vi "AUTOFLIM_Align.vi"(0 "Y Scan Center":dbl, 1 "X Scan Center":dbl, 2 "System no.":i32, 5 "Scan Termination":T1(ring), 7 "X":dbl, 9 "Y":dbl, 11 "error in (no error)":errorcluster, 12 "Z":dbl) -> (3 "Mesh out":dbl, 4 "Numeric 2":dbl, 6 "Numeric":dbl, 8 "Alignment Graph":dbl[][](array[numeric]), 10 "3D Line Graph":refnum<class "Base Datatype.lvclass">[](array[class]), 15 "error out":errorcluster)   [LabVIEW 2023]
uses:
  <vilib>/Native 3D Graph/classes/Base Datatype.lvclass
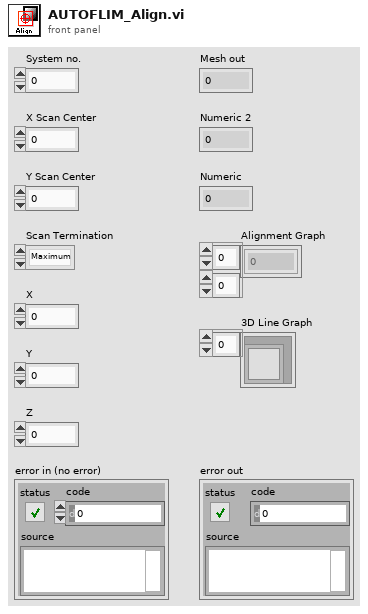
[diagram p1: front panel]
types:
  T1 = enum16{"Maximum", "End Position", "Center of scan"}
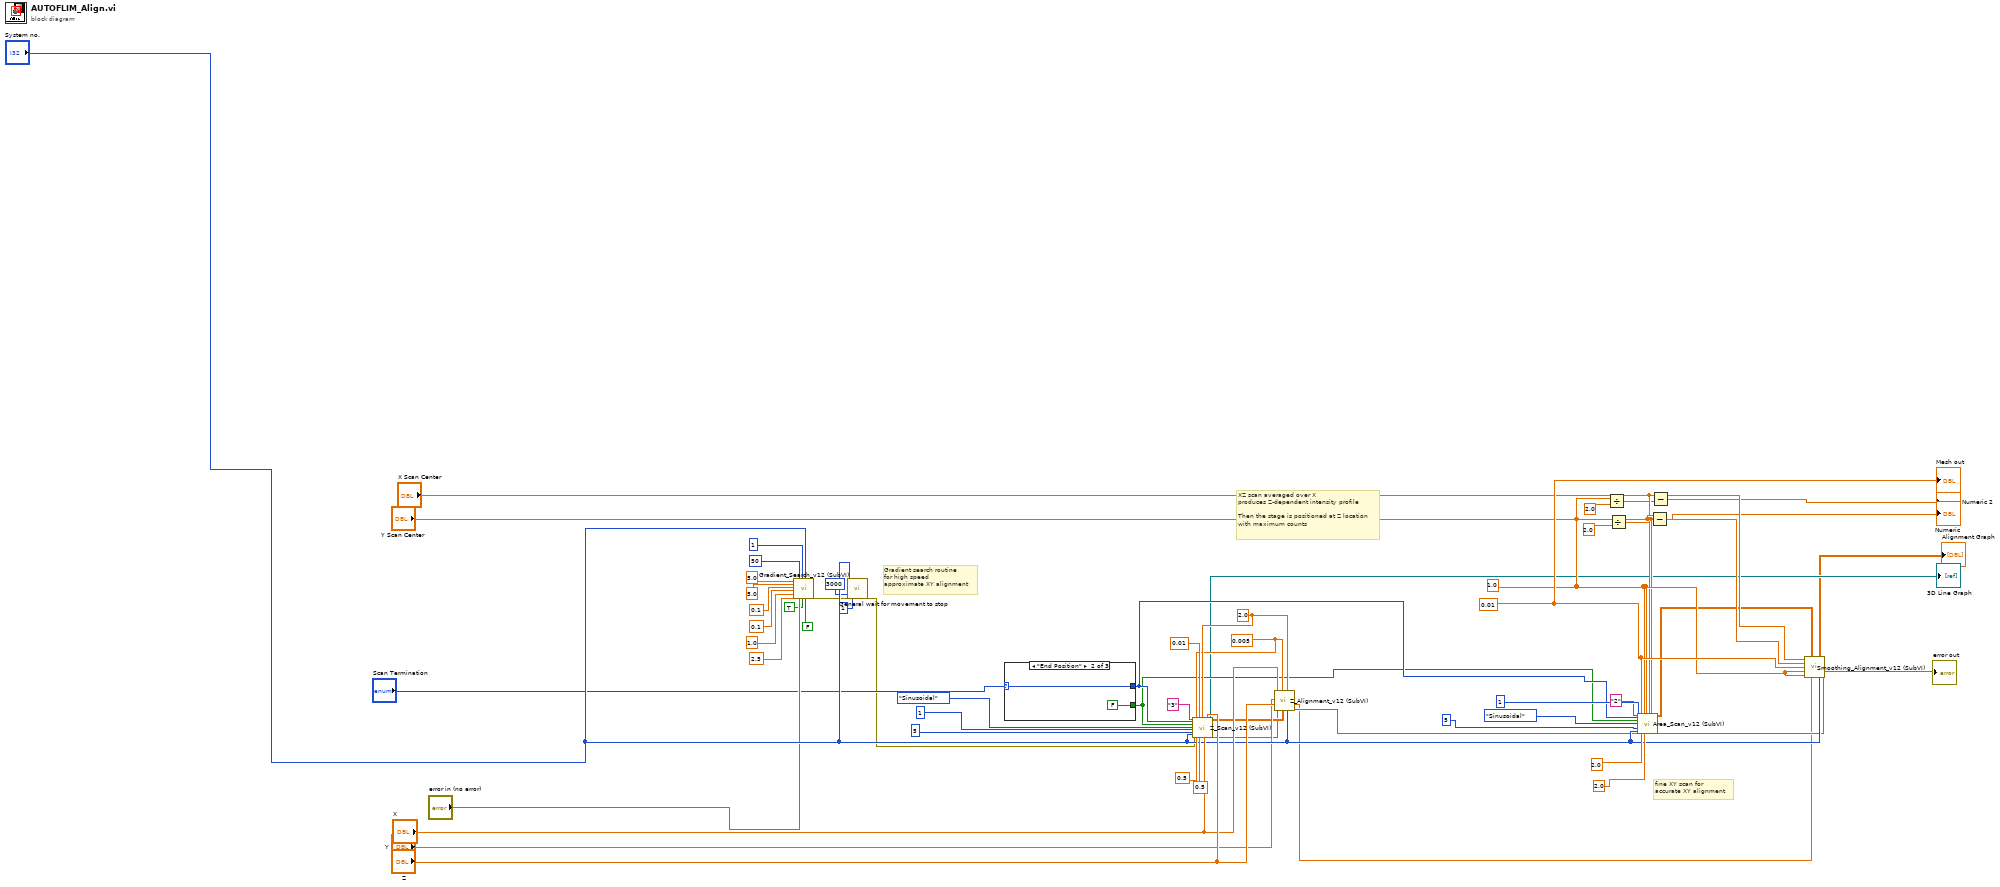
[diagram p0: block diagram]
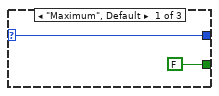
[diagram p2: hidden frame]
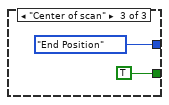
[diagram p3: hidden frame]
diagram:
  w54 = 0.01 ("Mesh in")
  w53 = 1.0 ("X Scan Range")
  w47 = 0.005 ("Z Mesh")
  w48 = 2.0 ("Z range")
  # "fine XY scan for\naccurate XY alignment"
  # "XZ scan averaged over X\nproduces Z-dependent intensity profile\n\nThen the stage is positioned at Z location\nwith maximum counts"
  # "Gradient search routine\nfor high speed\napproximate XY alignment"
  n1 = call "Gradient_Search_v12 (SubVI).vi"("Speed factor"=5.0, "Max velocity"=5.0, "ML"=0.1, "Min Radius"=0.1, "Max Radius"=1.0, "GS Frequency"=2.5, "Max. dir. changes"=50, "error in (no error)"="error in (no error)", "Analog Input"=1, "Run?"=TRUE, "System no."="System no.", "Tracking"=FALSE) -> ("error out"=w10:errorcluster)  [unwired: 7 in]
  n2 = call "General wait for movement to stop.vi"("System no."="System no.", "Additional wait time, ms"=3000, "error in"=w10, "Polling cycle \ntime, ms"=1) -> ("error out"=w9:errorcluster)  [unwired: 4 in, 11 out]
  n3 = case shown="\"End Position\"" "Scan Termination" {
    selector: "Scan Termination" -> [w58 w60 _]
    tunnel: [w58 w60 T1."End Position" ("Scan Termination")] -> w41
    tunnel: [FALSE FALSE TRUE] -> w40
    frame "Maximum", Default {
    }
    frame "End Position" {
    }
    frame "Center of scan" {
    }
  }
  n4 = call "Z_Scan_v12 (SubVI).vi"("Scan Axis"="3", "Scan Termination"=w41, "Center of Scan"=w40, "Scan Type"=enum16{"Sinusoidal", "Spiral"}."Sinusoidal", "Analog Input"=1, "Table rate"=5, "System no."="System no.", "error in (no error)"=w9, "Z Mesh"=w47, "Z-frequency"=0.5, "X Scan Range"=0.01, "Z-velocity"=0.5, "Z Scan Range"=w48, "X Scan Center"="X", "Z Scan Center"="Z") -> ("3D Line Graph"=→"3D Line Graph":refnum<class "Base Datatype.lvclass">[], "Intensity Graph"=w4:dbl[][], "error out"=w3:errorcluster)  [unwired: 8 in, 2 out]
  n5 = call "Z_Alignment_v12 (SubVI).vi"("System no."="System no.", "Z range"=w48, "Intensity Graph"=w4, "Z Mesh"=w47, "error in (no error)"=w3, "Z"="Z", "Y"="Y", "X"="X") -> ("error out"=w14:errorcluster, "Zout"=w1:dbl)  [unwired: 2 in]
  n6 = Divide(x=w53, y=2.0) -> (x/y=w20:dbl)
  n7 = Divide(x=w53, y=2.0) -> (x/y=w21:dbl)
  n8 = call "Area_Scan_v12 (SubVI).vi"("Step Axis"="2", "Scan Termination"=w41, "Center of Scan"=w40, "Scan Type"=enum16{"Sinusoidal", "Spiral"}."Sinusoidal", "Analog Input"=1, "Table rate"=5, "System no."="System no.", "error in (no error)"=w14, "Mesh in"=w54, "X-frequency"=2.0, "X Scan Range"=w53, "Y-velocity"=2.0 ("X-frequency"), "Y Scan Range"=w53, "X Scan Center"="X Scan Center", "Y Scan Center"="Y Scan Center") -> ("Intensity Graph"=w5:dbl[][], "error out"=w2:errorcluster)  [unwired: 8 in, 3 out]
  n9 = Subtract(x="Y Scan Center", y=w21) -> (x-y=→"Numeric":dbl)
  n10 = Subtract(x="X Scan Center", y=w20) -> (x-y=→"Numeric 2":dbl)
  n11 = call "Smoothing_Alignment_v12 (SubVI).vi"("X center"="X Scan Center", "Intensity Graph"=w5, "Y center"="Y Scan Center", "Mesh"=w54, "X Scan Range"=w53, "Y Scan Range"=w53, "Z"=w1, "System no."="System no.", "error in (no error)"=w2) -> ("Alignment Graph"=→"Alignment Graph":dbl[][], "error out"=→"error out":errorcluster)  [unwired: 5 in]
  "Mesh out" <- w54
